vi "loadHotLot.vi"() -> ()   [LabVIEW 2012]
uses:
  <vilib>/addons/database/Connection.llb/DB Tools Open Connec (Path).vi
  <vilib>/addons/database/NI_Database_API.lvlib
panel:
  in  "Cluster":cluster{"type":string, "desc":string}
  out "Value2":variant
  out "error out 2":errorcluster
  out "data":string[][](array[string])
  in  "end cell":string="h8192"
  in  "start cell":string="d5"
  in  "sheet#":i32=1
  out "error out":errorcluster
  in  "Excel._Worksheet":refnum<k7>
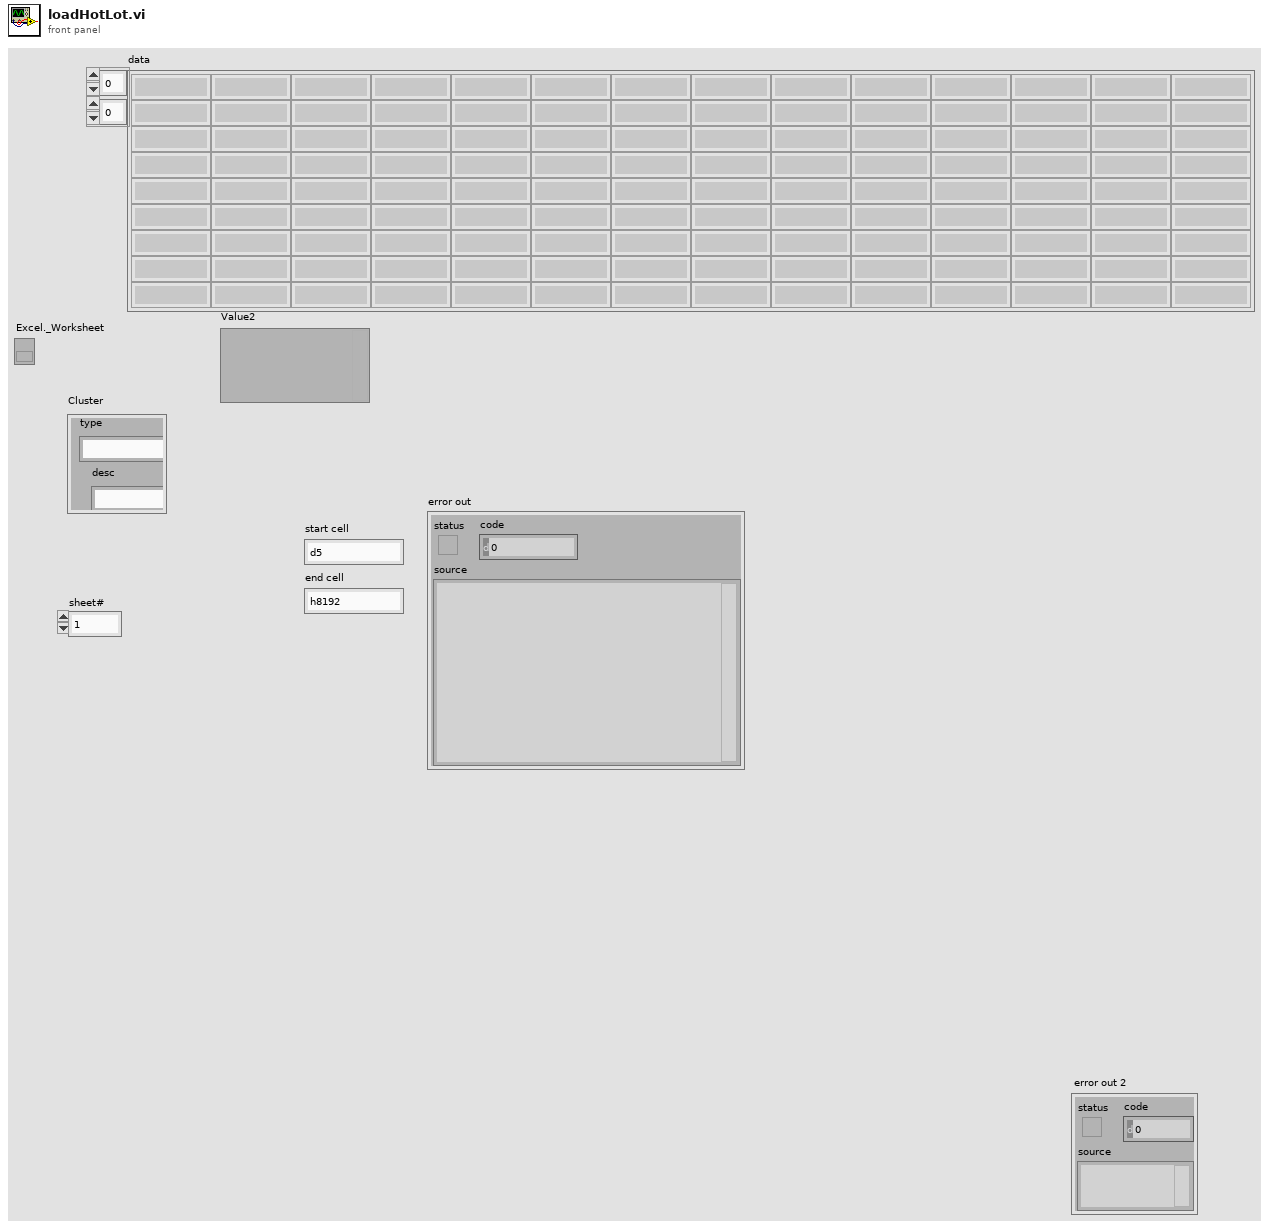
[diagram p1: front panel]
types:
  T1 = typedef "NI_Database_API.lvlib/Conn ObjectReference.ctl" = refnum<k1>
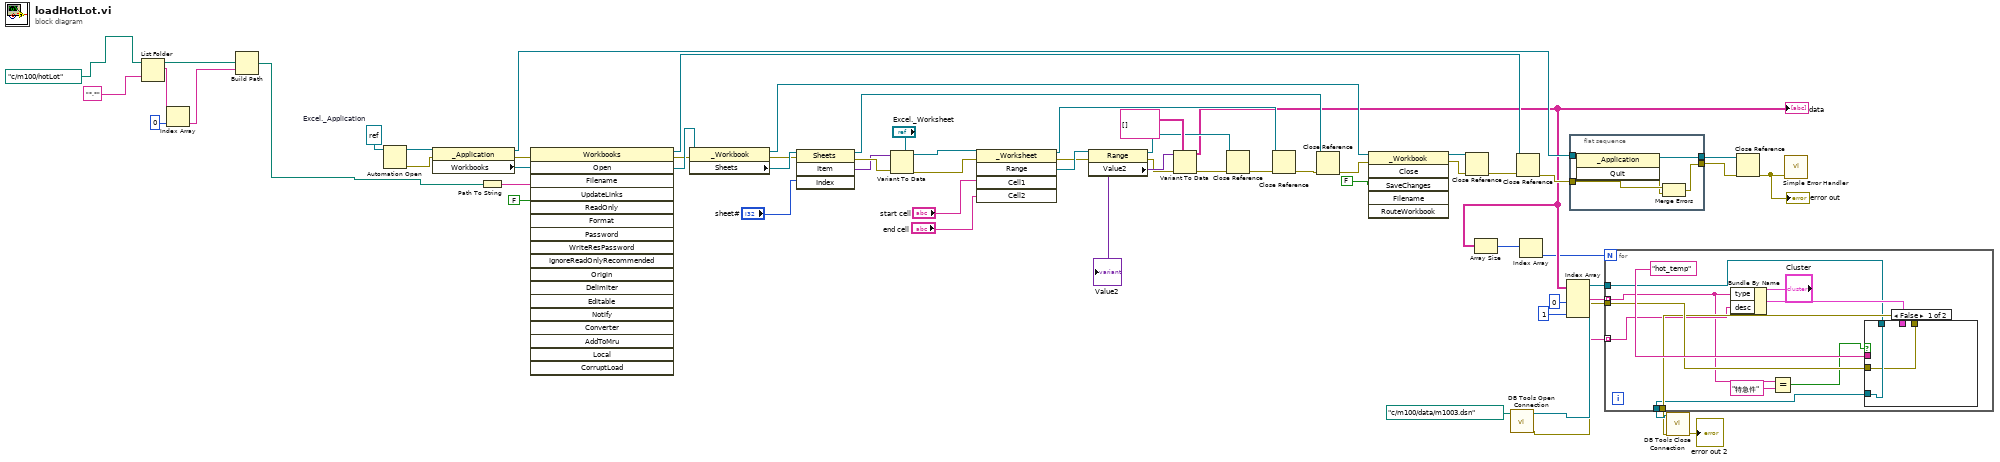
[diagram p0: block diagram]
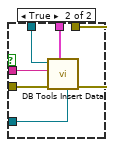
[diagram p2: hidden frame]
diagram:
  w25 = refnum<k7> refnum  # Excel._Application
  n1 = List Folder(path=path "c:/m100/hotLot", pattern="*.*") -> (path out=w61:path, filenames=w60:string[])  [unwired: 2 in, 2 out]
  n2 = Index Array(array=w60, index=0) -> (element=w59:string)
  n3 = Build Path(base path=w61, name or relative path=w59) -> (appended path=w15:path)
  n4 = Automation Open(Automation Refnum=w25) -> (Automation Refnum=w38:refnum<k7>, error out=w56:errorcluster)  [unwired: 3 in]
  n5 = property class="_Application"(reference=w38, error in=w56) -> (reference out=w28:refnum<k7>, error out=w54:errorcluster, "Workbooks"=w55:refnum<k7>)
  n6 = Path To String(path=w15) -> (string=w41:string)
  n7 = invoke class="Workbooks" method="Open"(reference=w55, error in=w54, "Filename"=w41, "ReadOnly"=FALSE) -> (reference out=w16:refnum<k7>, error out=w52:errorcluster, "Open"=w53:refnum<k7>)  [unwired: 14 in, 15 out]
  n8 = property class="_Workbook"(reference=w53, error in=w52) -> (reference out=w35:refnum<k7>, error out=w39:errorcluster, "Sheets"=w51:refnum<k7>)
  n9 = invoke class="Sheets" method="Item"(reference=w51, error in=w39, "Index"="sheet#") -> (reference out=w17:refnum<k7>, error out=w50:errorcluster, "Item"=w49:variant)  [unwired: 1 in, 1 out]
  n10 = Variant To Data(error in=w50, type="Excel._Worksheet", Variant=w49) -> (data=w48:refnum<k7>, error out=w47:errorcluster)
  n11 = invoke class="_Worksheet" method="Range"(reference=w48, error in=w47, "Cell1"="start cell", "Cell2"="end cell") -> (reference out=w19:refnum<k7>, error out=w45:errorcluster, "Range"=w46:refnum<k7>)  [unwired: 1 in, 2 out]
  n12 = property class="Range"(reference=w46, error in=w45) -> (reference out=w18:refnum<k7>, error out=w43:errorcluster, "Value2"=w44:variant)
  "Value2" <- w44
  n13 = Variant To Data(error in=w43, type=string[][] [], Variant=w44) -> (data=w5:string[][], error out=w42:errorcluster)
  "data" <- w5
  n14 = Close Reference(reference=w18, error in (no error)=w42) -> (error out=w37:errorcluster)
  n15 = Close Reference(reference=w19, error in (no error)=w37) -> (error out=w36:errorcluster)
  n16 = Close Reference(reference=w17, error in (no error)=w36) -> (error out=w34:errorcluster)
  n17 = invoke class="_Workbook" method="Close"(reference=w35, error in=w34, "SaveChanges"=FALSE) -> (reference out=w32:refnum<k7>, error out=w33:errorcluster)  [unwired: 3 in, 4 out]
  n18 = Close Reference(reference=w32, error in (no error)=w33) -> (error out=w31:errorcluster)
  n19 = Array Size(array=w5) -> (size(s)=w6:i32[])
  n20 = call-poly <vilib>:"DB Tools Open Connection.vi"("connection information"=path "c:/m100/data/m1003.dsn") -> ("error out"=w9:errorcluster, "connection reference"=w10:T1)  [unwired: 7 in]
  n21 = Close Reference(reference=w16, error in (no error)=w31) -> (error out=w30:errorcluster)
  n22 = Index Array(array=w6) -> (element=w4:i32)  [unwired: 1 in]
  n23 = Index Array(array=w5, index (col) #1=0 ("disabled index (col)"), index (col) #2=1 ("index (col)")) -> (element #1=w11:string[], element #2=w1:string[])  [unwired: 2 in]
  n24 = flat-sequence {
    tunnel: w30 -> [w65]
    tunnel: [w63] -> w29
    tunnel: w28 -> [w67]
    tunnel: [w66] -> w27
    frame #0 {
      n25 = invoke class="_Application" method="Quit"(reference=w67) -> (reference out=w66:refnum<k7>, error out=w64:errorcluster)  [unwired: 2 in, 1 out]
      n26 = Merge Errors(w65, w64) -> (w63:errorcluster)
    }
  }
  n27 = for {
    N: w4 -> [_]
    tunnel: w11 -> [w72] mode=indexing
    tunnel: w10 -> [w69]
    tunnel: w9 -> [w77]
    tunnel: [w68] -> w8
    tunnel: [w76] -> w7
    tunnel: w1 -> [w74] mode=indexing
    n28 = Bundle By Name(cluster="Cluster", "type"=w72, "desc"=w74) -> (w73:cluster{"type":string, "desc":string})
    n29 = Equal?(x=w72, y="特急件") -> (x = y?=w70:bool)
    n30 = case shown="False" w70 {
      tunnel: "hot_temp" ("table") -> [_ w86]
      tunnel: w77 -> [w79 w85]
      tunnel: [w79 w84] -> w76
      tunnel: w73 -> [_ w83]
      tunnel: w69 -> [w80 w82]
      tunnel: [w80 w81] -> w68
      frame False {
      }
      frame True {
        n31 = call <vilib>:"DB Tools Insert Data.vi"("data"=w83, "error in (no error)"=w85, "table"=w86, "connection reference"=w82) -> ("error out"=w84:errorcluster, "connection reference out"=w81:T1)  [unwired: 6 in]
      }
    }
  }
  n32 = call <vilib>:"DB Tools Close Connection.vi"("error in (no error)"=w7, "connection reference"=w8) -> ("error out"=→"error out 2":errorcluster)  [unwired: 5 in]
  n33 = Close Reference(reference=w27, error in (no error)=w29) -> (error out=w26:errorcluster)
  "error out" <- w26
  n34 = call <vilib>:"Simple Error Handler.vi"("error in (no error)"=w26) -> ()  [unwired: 4 in, 5 out]
